vi "SRV_Reset TCP Connection.vi"(8 "error in (no error)":errorcluster, 11 "IP address":string) -> (0 "error out":errorcluster, 3 "IP address dup":string)   [LabVIEW 2009]
doc: "Resets (opens, then closes) the SRV TCP connection.\n\n\nAuthor: Mike Schultz - Logic PD"
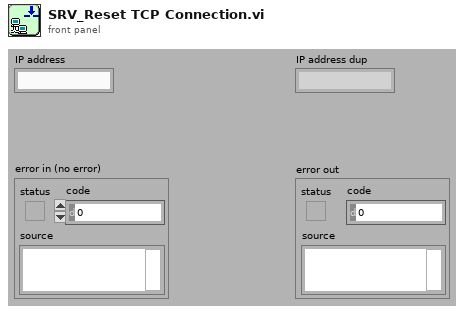
[diagram p1: front panel]
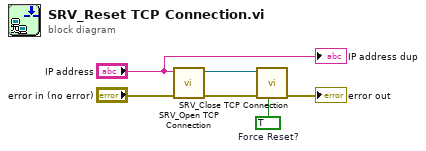
[diagram p0: block diagram]
diagram:
  w3 = TRUE  # Force Reset?
  n1 = call "SRV_Open TCP Connection.vi"("error in (no error)"="error in (no error)", "IP address"="IP address") -> ("error out"=w2:errorcluster, "connection ID"=w6:refnum<k5>)  [unwired: 8 in]
  n2 = call "SRV_Close TCP Connection.vi"("Force Reset? (F)"=w3, "error in"=w2, "connection ID"=w6) -> ("error out"=→"error out":errorcluster)  [unwired: 8 in]
  "IP address dup" <- "IP address"
